vi "flashV7.vi"() -> ()   [LabVIEW 2017]
panel:
  out "Out":u8 format="%.0x"
  out "字符串 2":string
  out "concatenated string":string
  in  "Register_Base_Address":u32=512 format="%x"
  in  "start":bool
  out "Current IP address":string
  in  "IP address list":string[](array[string])=["192.168.10.20", "192.168.10.22"]
  in  "回读":bool
  out "Current Progress":u32(slide)=3722240 scale=0.0..11418344.0
  out "error out":errorcluster={"status"=TRUE, "code"=4, "source"="Read from Binary File in flashV3.vi<APPEND>\nG:\\fpga_tdc\\FPGA\\TDC_2channel\\TOP.bin"}
  out "appended array":bool[](array[boolean])
  out "Process":u32=3722240
  in  "error in (no error)":errorcluster
  in  "Read (TRUE)":bool
  out "byte data":string
  out "Total size (in bytes)":i64=3722064
  in  "file path (use dialog)":path=path "G:/fpga_tdc/FPGA/SiTCP_410t/TDC_410t/TDC_410t.runs/impl_1/TOP.bin"
  # "FF80 0001 0000 0209 13"
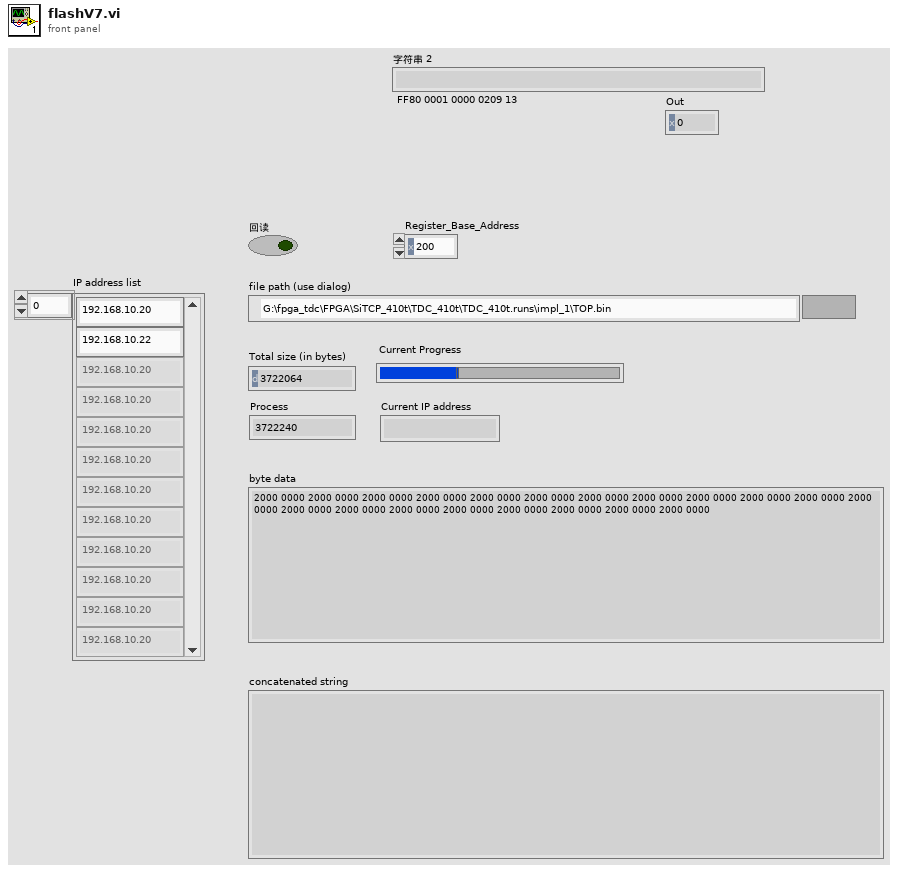
[diagram p1: front panel]
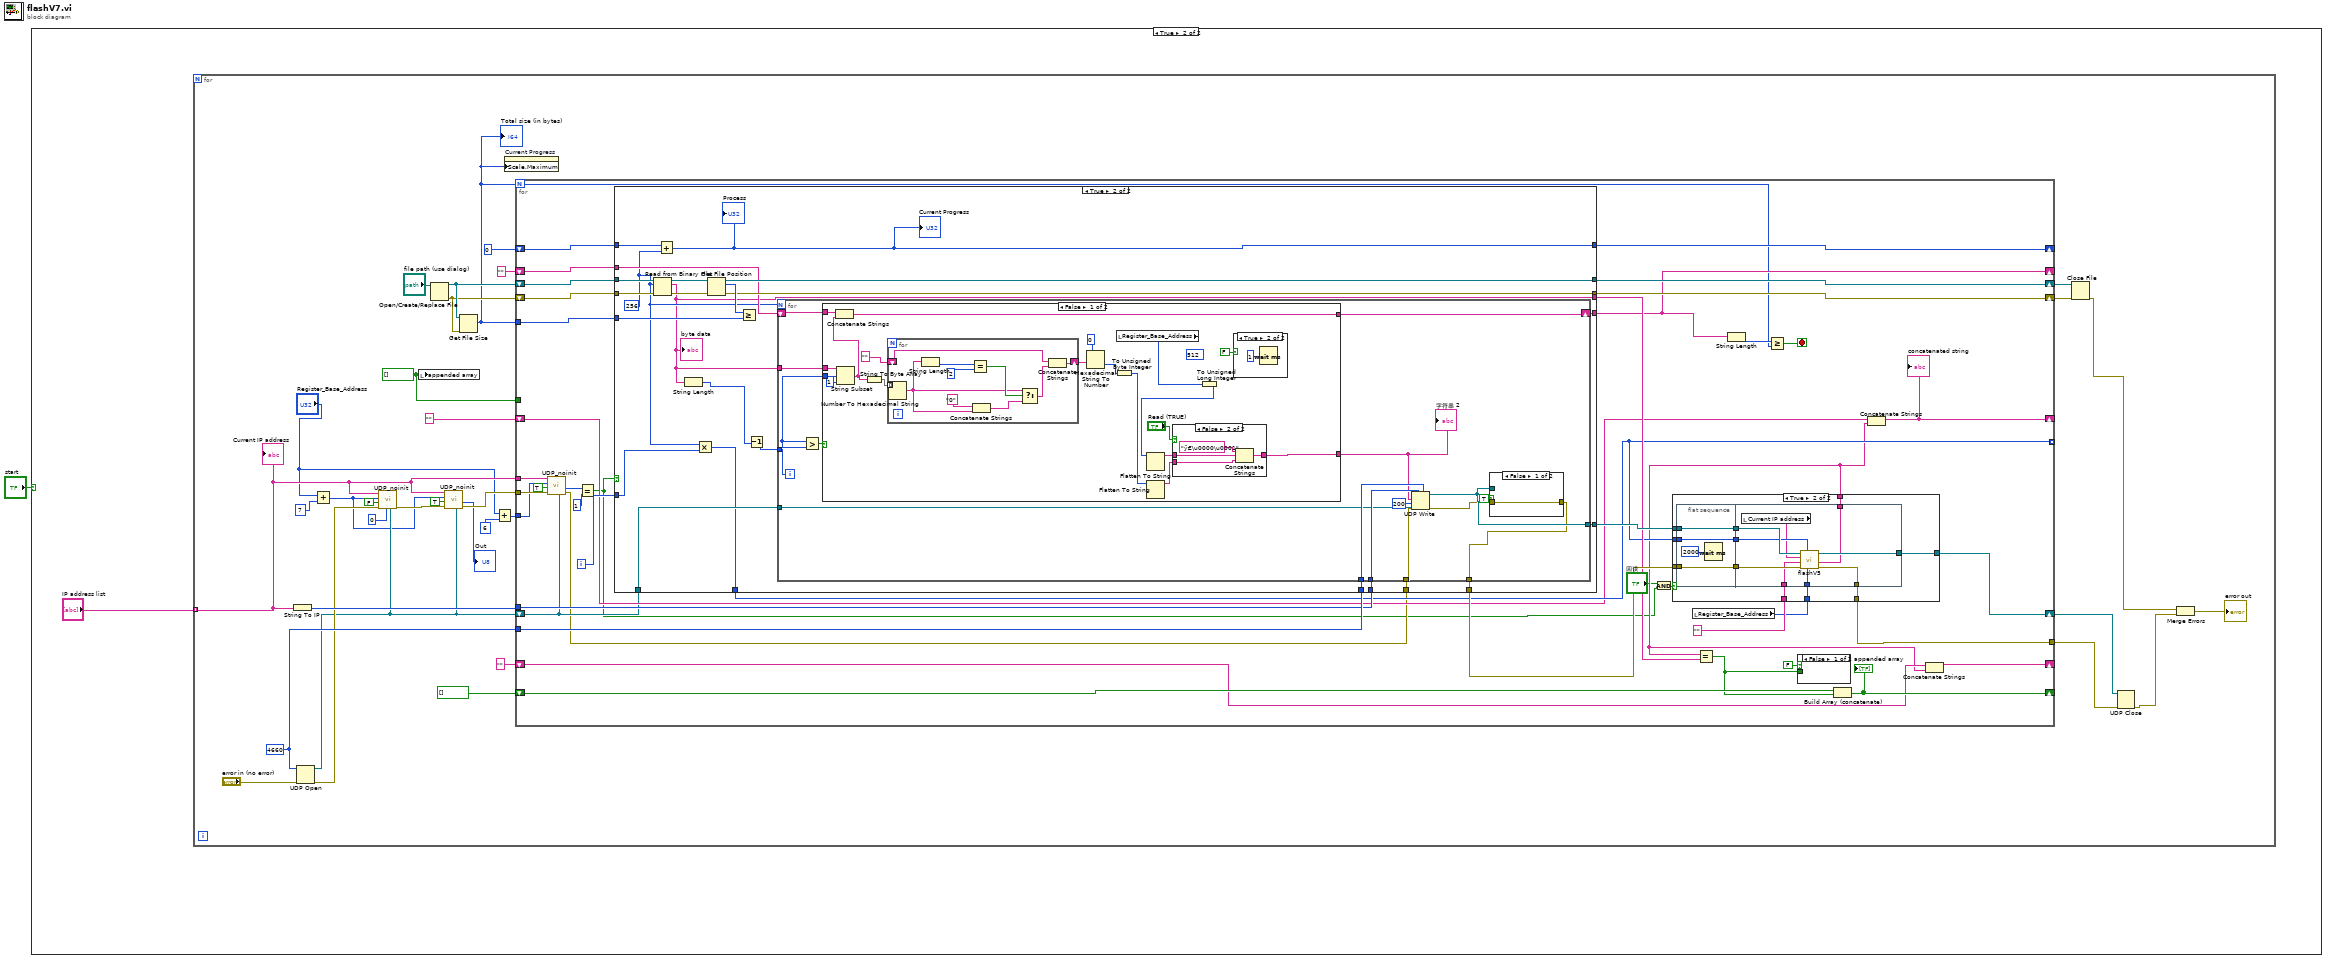
[diagram p0: block diagram]
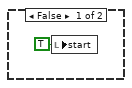
[diagram p2: hidden frame]
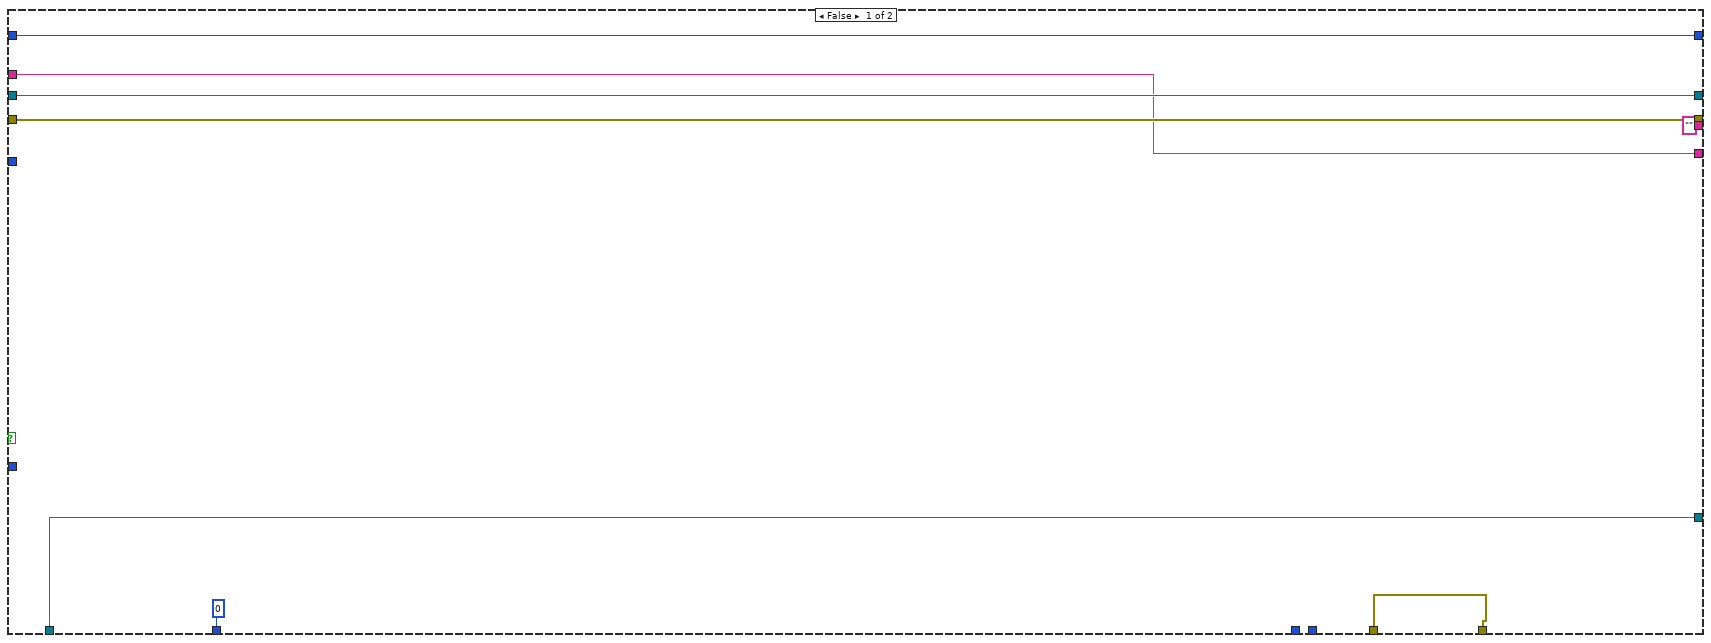
[diagram p3: hidden frame]
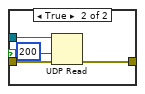
[diagram p4: hidden frame]
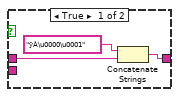
[diagram p5: hidden frame]
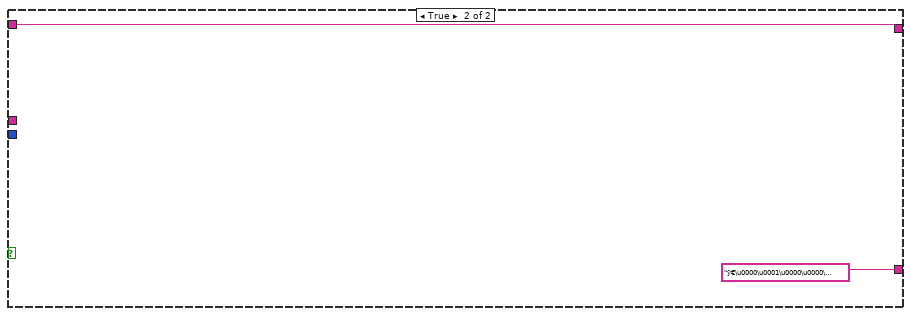
[diagram p7: hidden frame]
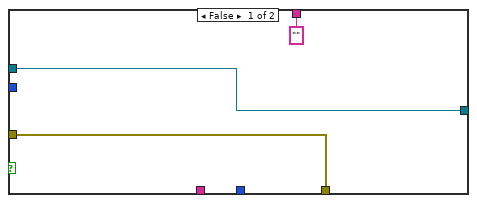
[diagram p8: hidden frame]
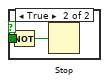
[diagram p9: hidden frame]
diagram:
  n1 = case shown="True" "start" {
    frame False {
      n2 = local write "start"(TRUE ("start")) -> ()
    }
    frame True {
      n3 = for {
        tunnel: "IP address list" -> [w19] mode=indexing
        w14 = bool[] [] ("appended array")
        w32 = u16 4660 ("UDP port")
        n4 = String To IP(1:w19) -> (0:w29:u32)
        n5 = UDP Open(8:"error in (no error)", 11:w32) -> (port=w17:refnum<k16>, 0:w21:errorcluster)  [unwired: 3 in, 1 out]
        n6 = Add(x="Register_Base_Address", y=u32 7 ("Address")) -> (x+y=w9:u32)
        n7 = call "UDP_noinit.vi"("connection ID"=w17, "In"=u8 0, "error in (no error)"=w21, "Read (TRUE)"=FALSE, "Address"=w9, "IP address"=w19) -> ("error out"=w20:errorcluster)  [unwired: 2 in, 2 out]
        n8 = local write "appended array"(w14) -> ()
        n9 = Open/Create/Replace File(file path (use dialog)="file path (use dialog)") -> (refnum out=w36:refnum<file>, error out=w35:errorcluster)  [unwired: 5 in, 1 out]
        n10 = call "UDP_noinit.vi"("connection ID"=w17, "error in (no error)"=w20, "Read (TRUE)"=TRUE, "Address"=w9, "IP address"=w19) -> ("error out"=w23:errorcluster, "Out"=→"Out":u8)  [unwired: 3 in, 1 out]
        n11 = Get File Size(file=w36, error in=w35) -> (size (in bytes)=w15:i64)  [unwired: 2 out]
        "Total size (in bytes)" <- w15
        n12 = Add(x="Register_Base_Address", y=u32 6 ("Address")) -> (x+y=w6:u32)
        n13 = property on="Current Progress" class="Slide (strict)"("Scale.Maximum"=w15) -> ()  [unwired: 2 in, 2 out]
        n14 = for {
          N: w15 -> [w57]
          tunnel: w15 -> [w78]
          shift-right: [w77] -> w34
          shift-left: w35 -> [w79]
          shift-right: [w76] -> w33
          shift-left: w36 -> [w80]
          shift-right: [w59] -> _
          shift-left: "" -> [w75]
          tunnel: w32 -> [w72]
          tunnel: [w67] -> w30
          tunnel: w29 -> [w71]
          shift-right: [w69] -> w31
          shift-left: w17 -> [w47]
          shift-right: [w73] -> _
          shift-left: u32 0 ("length (rest)") -> [w74]
          shift-right: [w64] -> _
          shift-left: bool[] [] -> [w62]
          tunnel: [w60] -> _ mode=indexing
          shift-right: [w55] -> _
          shift-left: "" -> [w54]
          tunnel: w19 -> [w52]
          tunnel: w23 -> [w46]
          shift-right: [w44] -> _
          shift-left: "" -> [w43]
          tunnel: w14 -> [_]
          tunnel: w6 -> [w39]
          i -> [w65]
          stop <- w56 stop-if-true
          n15 = call "UDP_noinit.vi"("connection ID"=w47, "error in (no error)"=w46, "Read (TRUE)"=TRUE, "Address"=w39, "IP address"=w52) -> ("error out"=w45:errorcluster, "Out"=w50:u8)  [unwired: 3 in, 1 out]
          n16 = Equal?(x=w50, y=u8 1) -> (x = y?=w41:bool)
          n17 = case shown="True" w41 {
            tunnel: w80 -> [w85 w112]
            tunnel: w79 -> [w86 w111]
            tunnel: w78 -> [_ w107]
            tunnel: [w86 w106] -> w77
            tunnel: [w85 w105] -> w76
            tunnel: w75 -> [w83 w104]
            tunnel: w74 -> [w84 w103]
            tunnel: [w84 w89] -> w73
            tunnel: w72 -> [_ w102]
            tunnel: w71 -> [_ w101]
            tunnel: w45 -> [w87 w100]
            tunnel: w47 -> [w88 w99]
            tunnel: [w88 w96] -> w70
            tunnel: [w87 w95] -> w68
            tunnel: w65 -> [_ w94]
            tunnel: ["" w92] -> w63
            tunnel: [0 w91] -> w60
            tunnel: [w83 w90] -> w59
            frame False {
            }
            frame True {
              w93 = 256 ("count (1)")
              n18 = Read from Binary File(8:w111, 10:w93, 11:w112) -> (0:w109:errorcluster, 2:w92:string, 3:w110:refnum<file>)  [unwired: 3 in, 1 out]
              "byte data" <- w92
              n19 = Add(x=w103, y=w93) -> (x+y=w89:u32)
              "Process" <- w89
              "Current Progress" <- w89
              n20 = String Length(string=w92) -> (length=w98:i32)
              n21 = Multiply(x=w93, y=w94) -> (x*y=w91:i32)
              n22 = Get File Position(4:w109, 7:w110) -> (0:w106:errorcluster, 2:w108:i64, 3:w105:refnum<file>)
              n23 = Greater Or Equal?(x=w108, y=w107) -> ()  [unwired: 1 out]
              n24 = Decrement(x=w98) -> (x-1=w97:i32)
              n25 = for {
                N: w93 -> [_]
                tunnel: w92 -> [w128]
                shift-right: [w126] -> w90
                shift-left: w104 -> [w127]
                tunnel: w102 -> [w125]
                tunnel: w101 -> [w124]
                tunnel: w100 -> [w123]
                tunnel: w99 -> [w117]
                tunnel: [w113] -> w95
                tunnel: [w116] -> w96
                tunnel: w97 -> [w120]
                i -> [w119]
                n26 = Greater?(x=w119, y=w120) -> (0:w121:bool)
                n27 = case shown="False" w121 {
                  tunnel: w128 -> [w145 _]
                  tunnel: w127 -> [w143 w171]
                  tunnel: [w142 w171] -> w126
                  tunnel: w119 -> [w136 _]
                  tunnel: [w135 "ÿ€\u0000\u0001\u0000\u0000\u0000@\u0000" ("字符串 2")] -> w118
                  frame False {
                    (unwired) u32 512 ("Address")
                    n28 = String Subset(string=w145, offset (0)=w136, length (rest)=1 ("length (rest)")) -> (substring=w141:string)
                    n29 = Concatenate Strings(w143, w141) -> (w142:string)
                    n30 = String To Byte Array(string=w141) -> (unsigned byte array=w151:u8[])
                    n31 = for {
                      shift-right: [w169] -> w150
                      shift-left: "" ("format string") -> [w166]
                      tunnel: w151 -> [w170] mode=indexing
                      n32 = Number To Hexadecimal String(2:w170) -> (0:w162:string)  [unwired: 1 in]
                      n33 = String Length(string=w162) -> (length=w168:i32)
                      n34 = Equal?(x=w168, y=2) -> (x = y?=w165:bool)
                      n35 = Concatenate Strings("0" ("format string"), w162) -> (w164:string)
                      n36 = Select(t=w162, s=w165, f=w164) -> (s? t:f=w161:string)
                      n37 = Concatenate Strings(w166, w161) -> (w169:string)
                    }
                    n38 = Hexadecimal String To Number(string=w150, default (0uL)=u64 0 ("default (0 U32)")) -> (number=w148:u64)  [unwired: 1 in, 1 out]
                    n39 = To Unsigned Byte Integer(number=w148) -> (unsigned 8bit integer=w147:u8)
                    n40 = local read "Register_Base_Address"() -> (w134:u32)
                    n41 = Flatten To String(anything=w147) -> (data string=w138:string)  [unwired: 3 in, 2 out]
                    n42 = To Unsigned Long Integer(number=w134) -> (unsigned 32bit integer=w146:u32)
                    n43 = Flatten To String(anything=w146) -> (data string=w139:string)  [unwired: 3 in, 2 out]
                    n44 = case shown="False" "Read (TRUE)" {
                      tunnel: [w154 w158] -> w135
                      tunnel: w139 -> [w153 w157]
                      tunnel: w138 -> [_ w156]
                      frame True {
                        n45 = Concatenate Strings("ÿÀ\u0000\u0001" ("initial string"), w153) -> (w154:string)
                      }
                      frame False {
                        n46 = Concatenate Strings("ÿ€\u0000\u0001" ("initial string"), w157, w156) -> (w158:string)
                      }
                    }
                    n47 = case shown="True" FALSE {
                      frame False {
                      }
                      frame True {
                        n48 = Wait (ms)(milliseconds to wait=u32 1) -> ()  [unwired: 1 out]
                      }
                    }
                  }
                  frame True {
                  }
                }
                "字符串 2" <- w118
                n49 = UDP Write(address=w124, port or service name=w125, connection ID=w117, data in=w118, 8:w123, 9:200 ("timeout ms (25000)")) -> (error out=w114:errorcluster, 3:w116:refnum<k16>)
                n50 = case shown="False" TRUE {
                  tunnel: w116 -> [_ w133]
                  tunnel: w114 -> [w129 w132]
                  tunnel: [w129 w131] -> w113
                  frame False {
                  }
                  frame True {
                    n51 = UDP Read(connection ID=w133, timeout ms (25000)=200, 8:w132) -> (error out=w131:errorcluster)  [unwired: 5 out]
                  }
                }
              }
            }
          }
          n52 = And(x="回读", y=w41) -> (x .and. y?=w48:bool)
          n53 = local read "Register_Base_Address"() -> (w38:u32)
          n54 = case shown="True" w48 {
            tunnel: w70 -> [w175 w183]
            tunnel: [w175 w182] -> w69
            tunnel: w68 -> [w174 w181]
            tunnel: [w174 w180] -> w67
            tunnel: "" ("empty") -> [_ w179]
            tunnel: w60 -> [_ w178]
            tunnel: ["" ("String") w177] -> w42
            tunnel: w38 -> [_ w176]
            frame False {
            }
            frame True {
              n55 = flat-sequence {
                tunnel: w178 -> [w188]
                tunnel: w181 -> [w189]
                tunnel: w183 -> [w190]
                tunnel: [w190] -> w186
                tunnel: [w189] -> w185
                tunnel: [w188] -> w184
                tunnel: [w196] -> w180
                tunnel: w179 -> [w195]
                tunnel: [w194] -> w177
                tunnel: w186 -> [w199]
                tunnel: w185 -> [w197]
                tunnel: w184 -> [w193]
                tunnel: [w198] -> w182
                tunnel: w176 -> [w191]
                frame #0 {
                  n56 = Wait (ms)(milliseconds to wait=u32 2000) -> ()  [unwired: 1 out]
                }
                frame #1 {
                  n57 = local read "Current IP address"() -> (w192:string)
                  n58 = call "flashV5.vi"("Register_Base_Address"=w191, "flash_base_address"=w193, "error in (no error)"=w197, "empty"=w195, "address"=w192, "connection ID"=w199) -> ("error out"=w196:errorcluster, "String"=w194:string, "connection ID 2"=w198:refnum<k16>)  [unwired: 2 in, 1 out]
                }
              }
            }
          }
          n59 = Equal?(x=w42, y=w63) -> (x = y?=w61:bool)
          n60 = String Length(string=w59) -> (length=w58:i32)
          n61 = Greater Or Equal?(x=w58, y=w57) -> (x >= y?=w56:bool)
          n62 = case shown="False" FALSE {
            tunnel: w61 -> [_ w200]
            frame False {
            }
            frame True {
              n63 = Not(x=w200) -> (.not. x?=w201:bool)
              n64 = Stop(stop? (T)=w201) -> ()
            }
          }
          n65 = Build Array (concatenate)(w62, w61) -> (w64:bool[])
          "appended array" <- w64
          n66 = Concatenate Strings(w54, w42) -> (w55:string)
          "concatenated string" <- w55
          n67 = Concatenate Strings(w43, w42) -> (w44:string)
        }
        n68 = Close File(refnum=w33, error in=w34) -> (error out=w13:errorcluster)  [unwired: 1 out]
        n69 = UDP Close(connection ID=w31, 8:w30) -> (error out=w12:errorcluster)  [unwired: 1 out]
        n70 = Merge Errors(w13, w12) -> (→"error out":errorcluster)
        "Current IP address" <- w19
      }
    }
  }
